vi "Event-Iterate.vi"(8 "error in (no error)":errorcluster, 10 "Data ref. in":refnum<data-value>, 11 "UI ref. in":refnum<data-value>) -> (0 "error out":errorcluster, 2 "Data ref.":refnum<data-value>, 3 "UI ref.":refnum<data-value>)   [LabVIEW 2013, in "CameraVision.lvlib" / "CV-UI.lvclass"]
uses:
  CV-UI.lvclass
  Main/CV-Main.lvclass
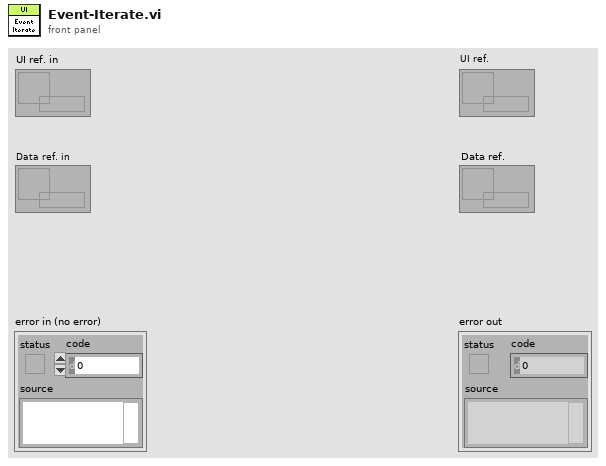
[diagram p1: front panel]
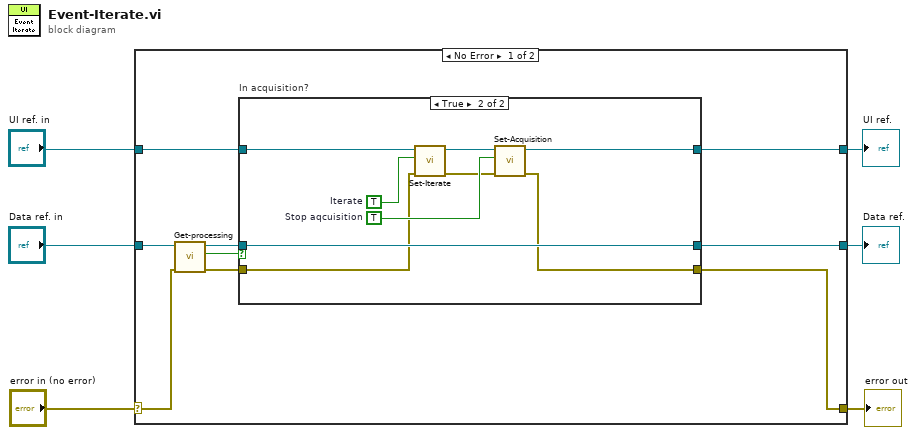
[diagram p0: block diagram]
diagram:
  n1 = case shown="No Error" "error in (no error)" {
    selector: "error in (no error)" -> [w9 w30]
    tunnel: [w7 w30] -> w5
    tunnel: [w12 w29] -> w3
    tunnel: "UI ref. in" -> [w10 w29]
    tunnel: "Data ref. in" -> [w15 w28]
    tunnel: [w11 w28] -> w1
    frame No Error {
      n2 = call "Get-processing.vi"("error in (no error)"=w9, "Data ref. in"=w15) -> ("error out"=w8:errorcluster, "Processing?"=w13:bool, "Data ref."=w14:refnum<data-value>)  [unwired: 7 in]
      n3 = case "In acquisition?" shown="True" w13 {
        tunnel: w10 -> [w17 w23]
        tunnel: w14 -> [w16 w26]
        tunnel: [w17 w27] -> w12
        tunnel: [w16 w26] -> w11
        tunnel: w8 -> [w18 w20]
        tunnel: [w18 w25] -> w7
        frame False {
        }
        frame True {
          w19 = TRUE  # Iterate
          w24 = TRUE  # Stop aqcuisition
          n4 = call "Set-Iterate.vi"("error in (no error)"=w20, "Iterate"=w19, "UI ref. in"=w23) -> ("error out"=w21:errorcluster, "UI ref."=w22:refnum<data-value>)  [unwired: 7 in]
          n5 = call "Set-Acquisition.vi"("error in (no error)"=w21, "Acquisition"=w24, "UI ref. in"=w22) -> ("error out"=w25:errorcluster, "UI ref."=w27:refnum<data-value>)  [unwired: 7 in]
        }
      }
    }
    frame Error {
    }
  }
  "error out" <- w5
  "Data ref." <- w1
  "UI ref." <- w3
